vi "Load Source Mouse.vi"(11 "Mouse Path":path) -> (0 "error out":errorcluster, 2 "Name":string, 3 "Mouse":refnum<class "Mouse.lvclass">)   [LabVIEW 2020, in "App.lvlib" / "MazeUI.lvclass"]
uses:
  MazeUI.lvclass
  Maze/Mouse/Mouse.lvclass
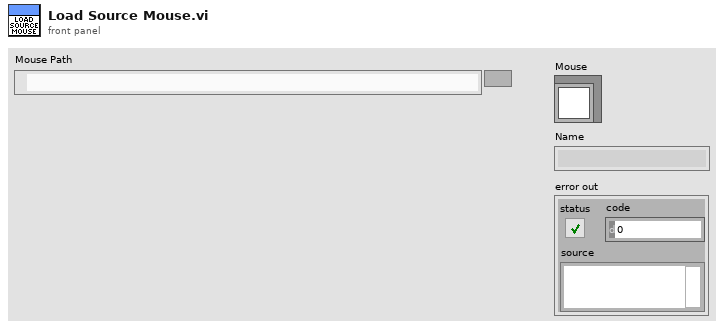
[diagram p1: front panel]
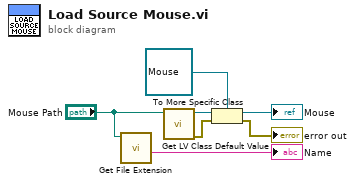
[diagram p0: block diagram]
diagram:
  n1 = call <vilib>:"Get File Extension.vi"("file"="Mouse Path") -> ("filename without extension"=→"Name":string)  [unwired: 6 in, 4 out]
  n2 = call <vilib>:"Get LV Class Default Value.vi"("class path"="Mouse Path") -> ("error out"=w5:errorcluster, "object"=w7:refnum<class>)  [unwired: 9 in]
  n3 = To More Specific Class(target class=refnum<class "Mouse.lvclass"> refnum ("Mouse"), reference=w7, error in=w5) -> (specific class reference=→"Mouse":refnum<class "Mouse.lvclass">, error out=→"error out":errorcluster)
